vi "Shared Get Object Pointer.vi"(11 "TreeNodeArray in":refnum<class "TreeNodeArray.lvclass">) -> (1 "Object Pointer":i64, 2 "Assigned object pointer?":bool, 3 "TreeNodeArray out":refnum<class "TreeNodeArray.lvclass">)   [LabVIEW 2013, in "MDSplus.lvlib" / "TreeNodeArray.lvclass"]
uses:
  <vilib>/MDSplus/Classes/TreeNodeArray_Class/TreeNodeArray.lvclass
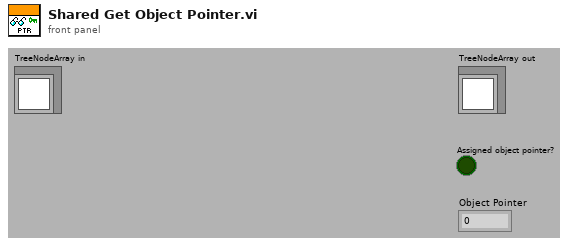
[diagram p1: front panel]
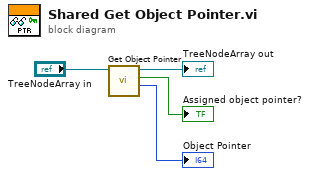
[diagram p0: block diagram]
diagram:
  n1 = call-dynamic "Get Object Pointer.vi"("TreeNodeArray in"="TreeNodeArray in") -> ("Object Pointer"=→"Object Pointer":i64, "Assigned object pointer?"=→"Assigned object pointer?":bool, "TreeNodeArray out"=→"TreeNodeArray out":refnum<class "TreeNodeArray.lvclass">)  [unwired: 8 in]
